vi "CounterEvent.vi"() -> ()   [LabVIEW 2020]
doc: "8-bit counter with buttons for user. Version with while loop and event structure. Comments in polish language."
panel:
  out "Num":bool[](array[boolean])
  out "TankOut":u8(slide) scale=0.0..255.0
  in  "Clear":bool
  out "NumOut":u8
  in  "Stop":bool
  in  "Dec":bool
  in  "Inc":bool
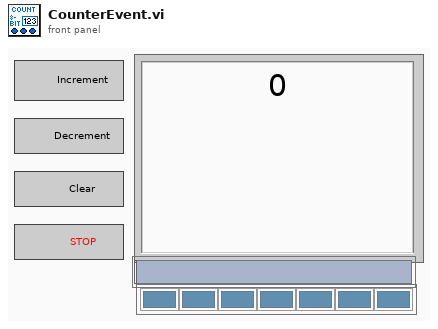
[diagram p1: front panel]
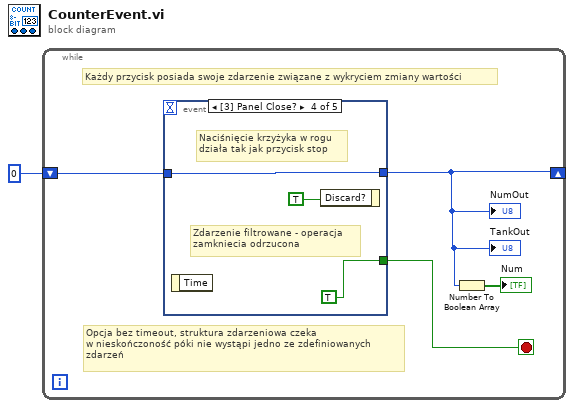
[diagram p0: block diagram]
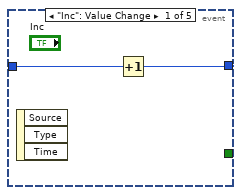
[diagram p2: hidden frame]
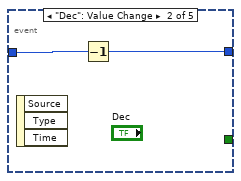
[diagram p3: hidden frame]
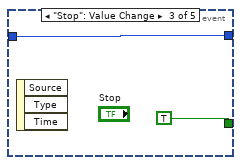
[diagram p4: hidden frame]
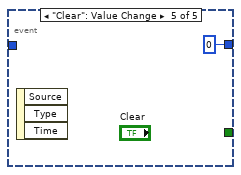
[diagram p5: hidden frame]
diagram:
  n1 = while {
    shift-right: [w3] -> _
    shift-left: u8 0 -> [w4]
    stop <- w2 stop-if-true
    # "Opcja bez timeout, struktura zdarzeniowa czeka\nw nieskończoność póki nie wystąpi jedno ze zdefiniowanych\nzdarzeń"
    # "Każdy przycisk posiada swoje zdarzenie związane z wykryciem zmiany wartości"
    n2 = event shown="[3] Panel Close?" {
      selector: _ -> [_ _ _ _ _]
      dyn-events: _ -> [_ _ _ _ _]
      timeout: _ -> [_ _ _ _ _]
      tunnel: w4 -> [w7 w9 w11 w13 _]
      tunnel: [w6 w8 w11 w13 u8 0] -> w3
      tunnel: [_ _ TRUE TRUE _] -> w2
      event "Inc": Value Change {
        n3 = event-data() -> ()  [unwired: 1 in, 3 out]
        n4 = Increment(x=w7) -> (x+1=w6:u8)
      }
      event "Dec": Value Change {
        n5 = event-data() -> ()  [unwired: 1 in, 3 out]
        n6 = Decrement(x=w9) -> (x-1=w8:u8)
      }
      event "Stop": Value Change {
        n7 = event-data() -> ()  [unwired: 1 in, 3 out]
      }
      event Panel Close? {
        # "Zdarzenie filtrowane - operacja \nzamkniecia odrzucona"
        # "Naciśnięcie krzyżyka w rogu\ndziała tak jak przycisk stop"
        n8 = event-data() -> ()  [unwired: 1 in, 1 out]
        n9 = event-data("Discard?"=TRUE) -> ()  [unwired: 1 in, 1 out]
      }
      event "Clear": Value Change {
        n10 = event-data() -> ()  [unwired: 1 in, 3 out]
      }
    }
    "NumOut" <- w3
    "TankOut" <- w3
    n11 = Number To Boolean Array(number=w3) -> (Boolean array=→"Num":bool[])
  }
